vi "ReadFile.vi"(8 "error in":errorcluster caption="错误输入", 9 "TransferMode":T1, 11 "FilePath":path) -> (0 "error out":errorcluster caption="错误输出", 1 "DataPack":string[](array[string]), 2 "FileName":string, 3 "FileNameSize":string, 4 "MD5":string, 5 "FileSize":string)   [LabVIEW 2013]
uses:
  TransferMode.ctl
panel:
  out "长度":i32
  out "PackageLen":i32
  out "LastPackDataLen":i32
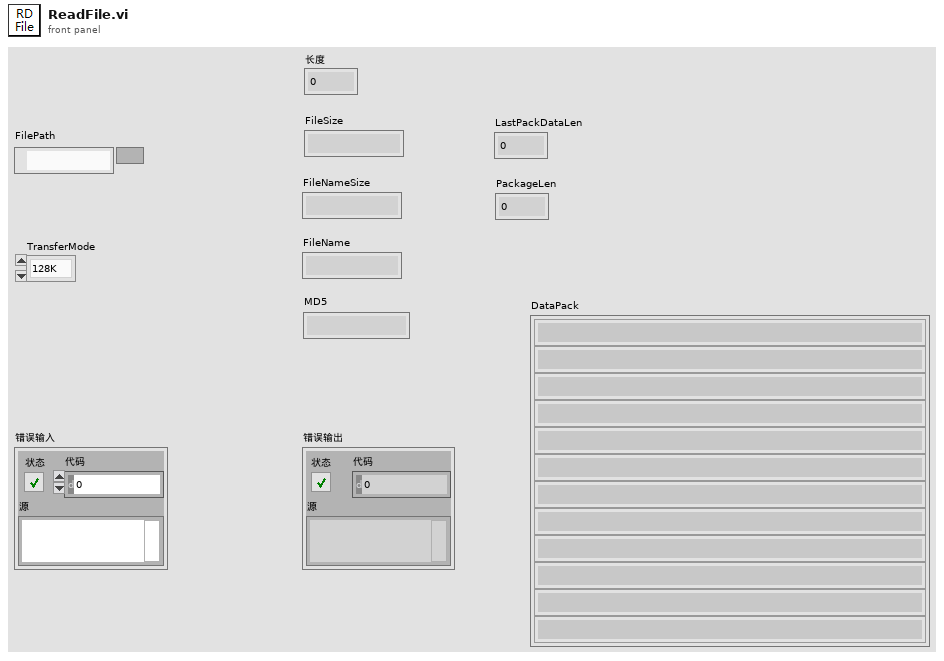
[diagram p1: front panel]
types:
  T1 = typedef "TransferMode.ctl" = enum16{"128K", "1024K"}
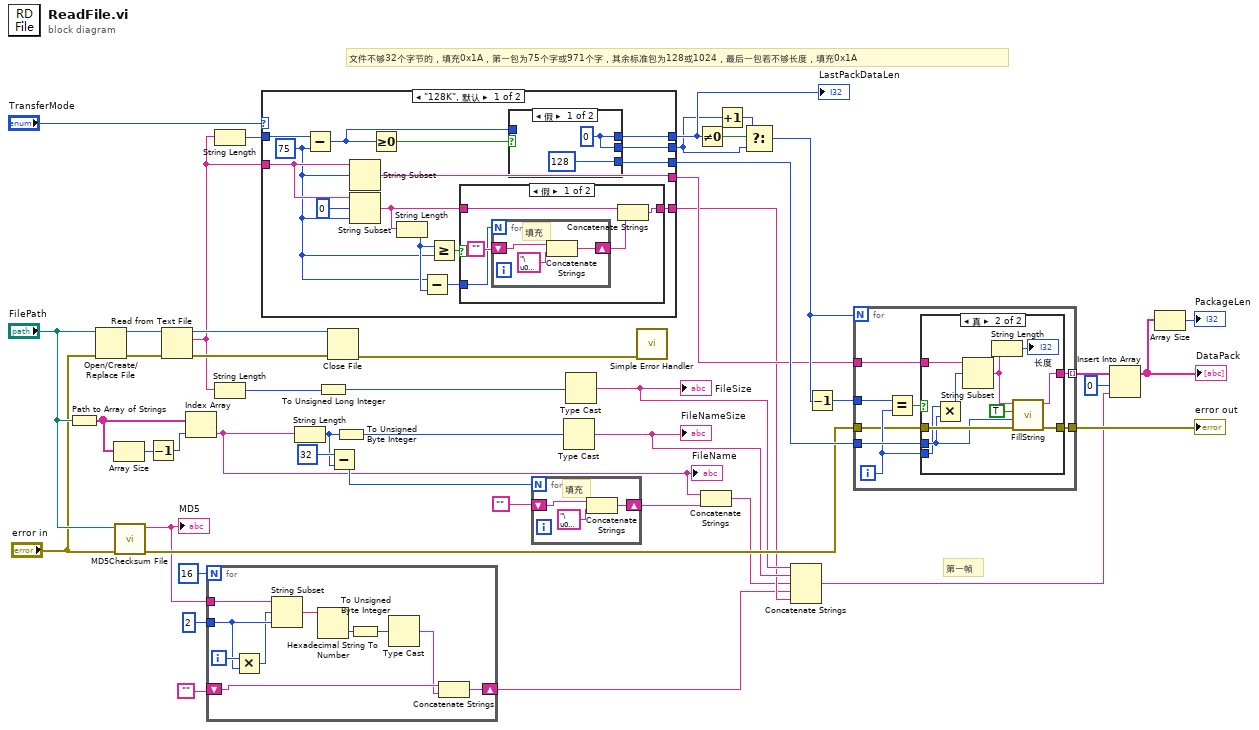
[diagram p0: block diagram]
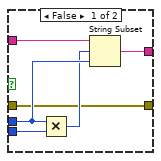
[diagram p2: hidden frame]
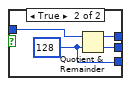
[diagram p3: hidden frame]
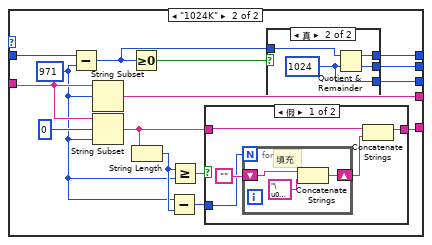
[diagram p5: hidden frame]
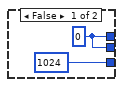
[diagram p6: hidden frame]
diagram:
  # "文件不够32个字节的，填充0x1A，第一包为75个字或971个字，其余标准包为128或1024，最后一包若不够长度，填充0x1A"
  # "第一帧"
  n1 = Path to Array of Strings(0:"FilePath") -> (2:w40:string[])  [unwired: 1 out]
  n2 = Open/Create/Replace File(file path (use dialog)="FilePath", error in="error in") -> (refnum out=w46:refnum<file>, error out=w45:errorcluster)  [unwired: 4 in, 1 out]
  n3 = Array Size(array=w40) -> (size(s)=w38:i32)
  n4 = call <vilib>:"MD5Checksum File.vi"("error in (no error)"="error in", "Path"="FilePath") -> ("error out"=w31:errorcluster, "MD5 message-digest"=w10:string)  [unwired: 8 in]
  "MD5" <- w10
  n5 = Decrement(x=w38) -> (x-1=w39:i32)
  n6 = Read from Text File(file (use dialog)=w46, error in=w45) -> (refnum out=w44:refnum<file>, text=w23:string, error out=w43:errorcluster)  [unwired: 2 in, 1 out]
  n7 = Index Array(array=w40, index=w39) -> (element=w2:string)
  "FileName" <- w2
  n8 = for {
    N: 16 -> [_]
    tunnel: w10 -> [w56]
    tunnel: 2 -> [w54]
    shift-right: [w49] -> w9
    shift-left: "" -> [w48]
    i -> [w55]
    n9 = Multiply(x=w55, y=w54) -> (x*y=w53:i32)
    n10 = String Subset(string=w56, offset (0)=w53, length (rest)=w54) -> (substring=w52:string)
    n11 = Hexadecimal String To Number(string=w52) -> (number=w50:u32)  [unwired: 2 in, 1 out]
    n12 = To Unsigned Byte Integer(number=w50) -> (unsigned 8bit integer=w51:u8)
    n13 = Type Cast(x=w51) -> (*(type *) &x=w47:string)  [unwired: 1 in]
    n14 = Concatenate Strings(w48, w47) -> (w49:string)
  }
  n15 = String Length(string=w23) -> (length=w34:i32)
  n16 = String Length(string=w23) -> (length=w42:i32)
  n17 = case shown="\"128K\", 默认" "TransferMode" {
    tunnel: w34 -> [w71 w101]
    tunnel: [w70 w90] -> w1
    tunnel: [w69 w91] -> w24
    tunnel: [w68 w89] -> w33
    tunnel: w23 -> [w66 w99]
    tunnel: [w67 w100] -> w22
    tunnel: [w62 w97] -> w18
    frame "128K", Default {
      w57 = 75 ("y")
      n18 = Subtract(x=w71, y=w57) -> (x-y=w58:i32)
      n19 = String Subset(string=w66, offset (0)=w57) -> (substring=w67:string)  [unwired: 1 in]
      n20 = String Subset(string=w66, offset (0)=0 ("y"), length (rest)=w57) -> (substring=w63:string)
      n21 = Greater Or Equal To 0?(x=w58) -> (x >= 0?=w59:bool)
      n22 = String Length(string=w63) -> (length=w61:i32)
      n23 = Subtract(x=w57, y=w61) -> (x-y=w60:i32)
      n24 = Greater Or Equal?(x=w61, y=w57) -> (x >= y?=w64:bool)
      n25 = case shown="假" w64 {
        tunnel: w63 -> [w79 w86]
        tunnel: [w80 w86] -> w62
        tunnel: w60 -> [w81 _]
        frame False {
          n26 = for {
            N: w81 -> [_]
            shift-right: [w84] -> w78
            shift-left: "" -> [w83]
            # "填充"
            n27 = Concatenate Strings(w83, "\u001a") -> (w84:string)
          }
          n28 = Concatenate Strings(w79, w78) -> (w80:string)
        }
        frame True {
        }
      }
      n29 = case shown="假" w59 {
        tunnel: [w72 w77] -> w70
        tunnel: [w72 w76] -> w69
        tunnel: [128 ("y") w75] -> w68
        tunnel: w58 -> [_ w74]
        frame False {
          w72 = 0
        }
        frame True {
          w75 = 128 ("y")
          n30 = Quotient & Remainder(x=w74, y=w75) -> (x-y*floor(x/y)=w76:i32, floor(x/y)=w77:i32)
        }
      }
    }
    frame "1024K" {
      w87 = 971
      n31 = Subtract(x=w101, y=w87) -> (x-y=w88:i32)
      n32 = String Subset(string=w99, offset (0)=w87) -> (substring=w100:string)  [unwired: 1 in]
      n33 = String Subset(string=w99, offset (0)=0, length (rest)=w87) -> (substring=w96:string)
      n34 = Greater Or Equal To 0?(x=w88) -> (x >= 0?=w92:bool)
      n35 = String Length(string=w96) -> (length=w93:i32)
      n36 = Subtract(x=w87, y=w93) -> (x-y=w94:i32)
      n37 = Greater Or Equal?(x=w93, y=w87) -> (x >= y?=w95:bool)
      n38 = case shown="假" w95 {
        tunnel: w96 -> [w110 w116]
        tunnel: [w108 w116] -> w97
        tunnel: w94 -> [w111 _]
        frame False {
          n39 = for {
            N: w111 -> [_]
            shift-right: [w114] -> w109
            shift-left: "" -> [w113]
            # "填充"
            n40 = Concatenate Strings(w113, "\u001a") -> (w114:string)
          }
          n41 = Concatenate Strings(w110, w109) -> (w108:string)
        }
        frame True {
        }
      }
      n42 = case shown="真" w92 {
        tunnel: [w102 w107] -> w90
        tunnel: [w102 w106] -> w91
        tunnel: [1024 ("y") w105] -> w89
        tunnel: w88 -> [_ w104]
        frame False {
          w102 = 0
        }
        frame True {
          w105 = 1024 ("y")
          n43 = Quotient & Remainder(x=w104, y=w105) -> (x-y*floor(x/y)=w106:i32, floor(x/y)=w107:i32)
        }
      }
    }
  }
  "LastPackDataLen" <- w24
  n44 = String Length(string=w2) -> (length=w7:i32)
  n45 = To Unsigned Long Integer(number=w42) -> (unsigned 32bit integer=w41:u32)
  n46 = Close File(refnum=w44, error in=w43) -> (error out=w28:errorcluster)  [unwired: 1 out]
  n47 = Subtract(x=32, y=w7) -> (x-y=w6:i32)
  n48 = To Unsigned Byte Integer(number=w7) -> (unsigned 8bit integer=w37:u8)
  n49 = for {
    N: w6 -> [_]
    shift-right: [w118] -> w4
    shift-left: "" -> [w117]
    # "填充"
    n50 = Concatenate Strings(w117, "\u001a") -> (w118:string)
  }
  n51 = Type Cast(x=w37) -> (*(type *) &x=w19:string)  [unwired: 1 in]
  "FileNameSize" <- w19
  n52 = Type Cast(x=w41) -> (*(type *) &x=w20:string)  [unwired: 1 in]
  "FileSize" <- w20
  n53 = call <vilib>:"Simple Error Handler.vi"("error in (no error)"=w28) -> ()  [unwired: 4 in, 5 out]
  n54 = Not Equal To 0?(x=w24) -> (x != 0?=w27:bool)
  n55 = Concatenate Strings(w2, w4) -> (w3:string)
  n56 = Increment(x=w1) -> (x+1=w26:i32)
  n57 = Select(t=w26, s=w27, f=w1) -> (s? t:f=w25:i32)
  n58 = Concatenate Strings(w20, w19, w3, w9, w18) -> (w14:string)
  n59 = Decrement(x=w25) -> (x-1=w32:i32)
  n60 = for {
    N: w25 -> [_]
    tunnel: w33 -> [w126]
    tunnel: w22 -> [w127]
    tunnel: w32 -> [w124]
    tunnel: [w122] -> w16 mode=indexing
    tunnel: w31 -> [w121]
    tunnel: [w120] -> w30
    i -> [w123]
    n61 = Equal?(x=w124, y=w123) -> (x = y?=w125:bool)
    n62 = case shown="真" w125 {
      tunnel: w123 -> [w133 w137]
      tunnel: w127 -> [w132 w143]
      tunnel: w126 -> [w131 w138]
      tunnel: [w129 w142] -> w122
      tunnel: w121 -> [w128 w141]
      tunnel: [w128 w140] -> w120
      frame False {
        n63 = Multiply(x=w131, y=w133) -> (x*y=w130:i32)
        n64 = String Subset(string=w132, offset (0)=w130, length (rest)=w131) -> (substring=w129:string)
      }
      frame True {
        n65 = Multiply(x=w137, y=w138) -> (x*y=w136:i32)
        n66 = String Subset(string=w143, offset (0)=w136) -> (substring=w135:string)  [unwired: 1 in]
        n67 = String Length(string=w135) -> (length=→"长度":i32)
        n68 = call "FillString.vi"("error in"=w141, "PackLen"=w138, "Fill?"=TRUE, "StringIn"=w135) -> ("error out"=w140:errorcluster, "StringOut"=w142:string)  [unwired: 6 in]
      }
    }
  }
  "error out" <- w30
  n69 = Insert Into Array(array=w16, index=0 ("索引"), new element=w14) -> (w15:string[])
  "DataPack" <- w15
  n70 = Array Size(array=w15) -> (size(s)=→"PackageLen":i32)
